vi "Run.vi"(11 "error in (no error)":errorcluster) -> (15 "error out":errorcluster)   [LabVIEW 2016, in "TimerTest.lvlib"]
doc: "Run all tests in library"
uses:
  TimerTest.lvlib
  Drona.lvlib
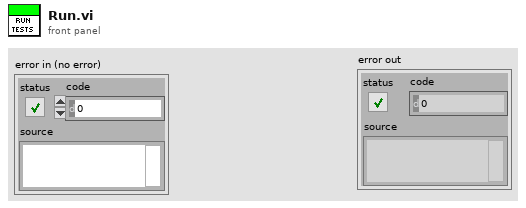
[diagram p1: front panel]
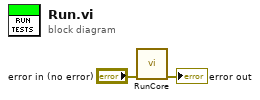
[diagram p0: block diagram]
diagram:
  n1 = call "RunCore.vi"("error in"="error in (no error)") -> ("error out"=→"error out":errorcluster)  [unwired: 10 in]
